vi "Draw Tree.vi"(10 "Tree Control Items":T1(array[cluster]), 11 "TreeControl in":refnum<vi>) -> (0 "error out":errorcluster)   [LabVIEW 2020, in "Panther Dashboard.lvlib"]
uses:
  Panther Dashboard.lvlib
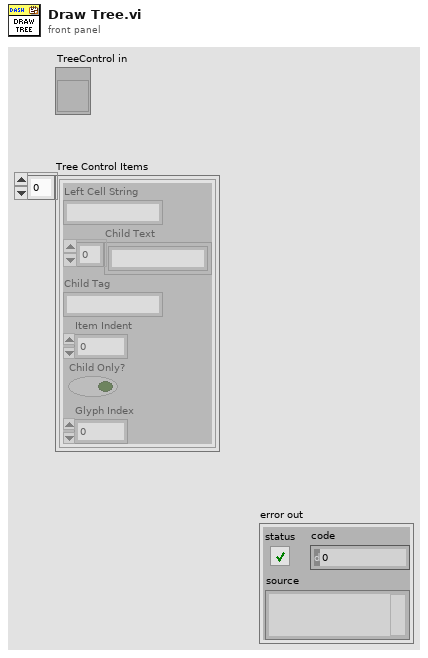
[diagram p1: front panel]
types:
  T1 = cluster{"Left Cell String":string, "Child Text":string[], "Child Tag":string, "Item Indent":i32, "Child Only?":bool, "Glyph Index":i32}[]
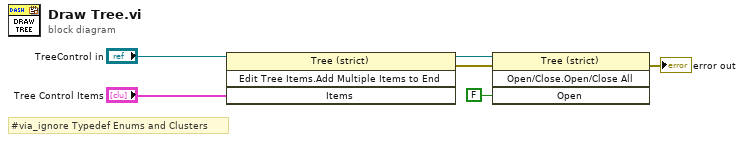
[diagram p0: block diagram]
diagram:
  # "#via_ignore Typedef Enums and Clusters"
  n1 = invoke on="Invoke Node" class="Tree (strict)" method="Edit Tree Items.Add Multiple Items to End"(reference="TreeControl in", "Items"="Tree Control Items") -> (reference out=w2:refnum<vi>, error out=w6:errorcluster)  [unwired: 2 in, 2 out]
  n2 = invoke class="Tree (strict)" method="Open/Close.Open/Close All"(reference=w2, error in=w6, "Open"=FALSE ("Open?")) -> (error out=→"error out":errorcluster)  [unwired: 1 in, 3 out]
